vi "UseDefault.vi"(6 "error in":errorcluster, 9 "Terminal in":refnum<class "Terminal.lvclass">) -> (0 "error out":errorcluster, 3 "Terminal out":refnum<class "Terminal.lvclass">, 4 "Use Default":bool)   [LabVIEW 2014, in "Terminal.lvclass"]
uses:
  Terminal.lvclass
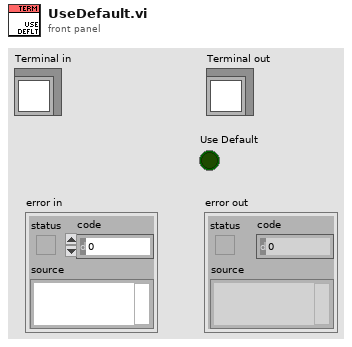
[diagram p1: front panel]
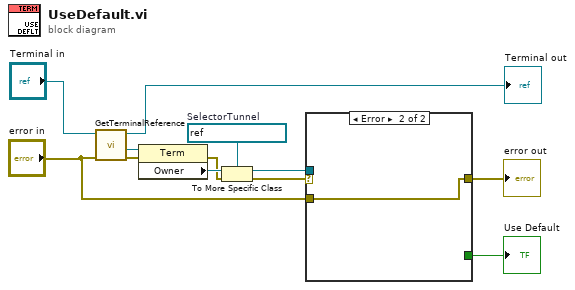
[diagram p0: block diagram]
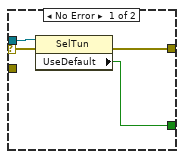
[diagram p2: hidden frame]
diagram:
  w10 = refnum<vi> refnum  # SelectorTunnel
  n1 = call "GetTerminalReference.vi"("error in"="error in", "Terminal in"="Terminal in") -> ("error out"=w7:errorcluster, "reference"=w8:refnum<vi>, "Terminal out"=→"Terminal out":refnum<class "Terminal.lvclass">)  [unwired: 7 in]
  n2 = property class="Term"(reference=w8, error in=w7) -> (error out=w3:errorcluster, "Owner"=w9:refnum<vi>)  [unwired: 1 out]
  n3 = To More Specific Class(target class=w10, reference=w9, error in=w3) -> (specific class reference=w11:refnum<vi>, error out=w6:errorcluster)
  n4 = case shown="Error" w6 {
    selector: w6 -> [w15 _]
    tunnel: w11 -> [w16 _]
    tunnel: [w14 _] -> w5
    tunnel: [w13 w17] -> w1
    tunnel: "error in" -> [_ w17]
    frame No Error {
      n5 = property class="SelTun"(reference=w16, error in=w15) -> (error out=w13:errorcluster, "UseDefault"=w14:bool)  [unwired: 1 out]
    }
    frame Error {
    }
  }
  "error out" <- w1
  "Use Default" <- w5
